vi "UpdateData.vi"(9 "Data in 2":dbl[](array[numeric]), 10 "Data in":dbl[](array[numeric]), 11 "output cluster 2":T1) -> (1 "Integral X":dbl[](array[numeric]), 2 "Data out":dbl[][](array[numeric]), 3 "output cluster 3":T1, 4 "data out 2":dbl[](array[numeric]), 5 "size(s)":i32)   [LabVIEW 2016]
doc: "concatenates previuos data to new data and outputs the current graph data"
uses:
  <vilib>/Analysis/NI_AALPro.lvlib
  LoopData.ctl
  EK-P4/EK-P4.lvclass
panel:
  out "size(s) 3":i32
  out "size(s) 5":i32
  out "size(s) 4":i32
  out "size(s) 2":i32[](array[numeric])
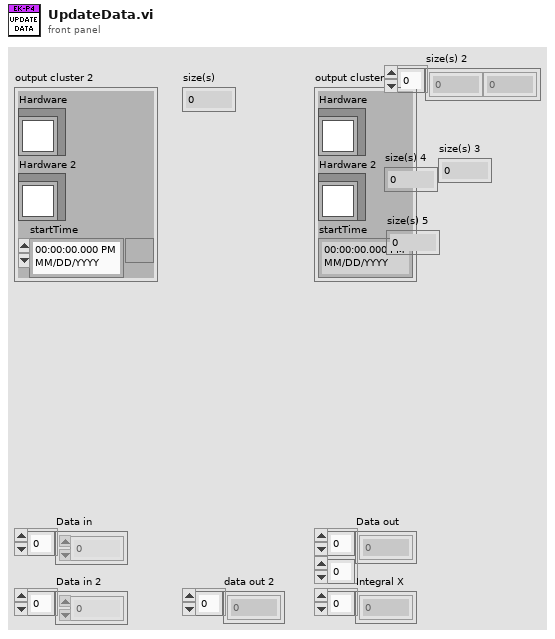
[diagram p1: front panel]
types:
  T1 = typedef "LoopData.ctl" = cluster{"Hardware":refnum<class "EK-P4.lvclass">, "Hardware 2":refnum<class "EK-P4.lvclass">, "startTime":timestamp}
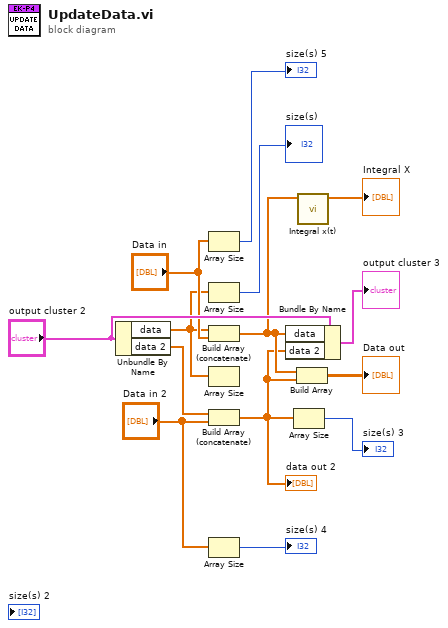
[diagram p0: block diagram]
diagram:
  n1 = Unbundle By Name("output cluster 2") -> ("data"=w5:dbl[], "data 2"=w7:dbl[])
  n2 = Array Size(array="Data in") -> (size(s)=→"size(s) 5":i32)
  n3 = Array Size(array=w5) -> (size(s)=→"size(s)":i32)
  n4 = Build Array (concatenate)(w5, "Data in") -> (w3:dbl[])
  n5 = Array Size(array=w5) -> ()  [unwired: 1 out]
  n6 = Build Array (concatenate)(w7, "Data in 2") -> (w2:dbl[])
  "data out 2" <- w2
  n7 = Array Size(array="Data in 2") -> (size(s)=→"size(s) 4":i32)
  n8 = Bundle By Name(cluster="output cluster 2", "data"=w3, "data 2"=w2) -> (→"output cluster 3":T1)
  n9 = Array Size(array=w2) -> (size(s)=→"size(s) 3":i32)
  n10 = Build Array(w3, w2) -> (→"Data out":dbl[][])
  n11 = call <vilib>:"Integral x(t).vi"("X"=w3) -> ("Integral X"=→"Integral X":dbl[])  [unwired: 9 in, 1 out]
